vi "Interfaz comunicación chaskas.vi"() -> ()   [LabVIEW 2018]
uses:
  <vilib>/Instr/_visa.llb/VISA Configure Serial Port (Instr).vi
panel:
  out "String":string
  in  "string":string
  in  "Información serial":string
  in  "Interfaz":T1(tab)
  out "Ventana de avisos":string
  out "Nieve disponible":bool
  out "Administrador":bool
  in  "Cerrar Sesión":bool
  in  "Contraseña":string
  out "Usuario actual":string
  in  "Login 2":bool
  in  "Pedido":bool
  in  "Chocolate":bool
  in  "Cereal1":bool
  in  "Cereal 2":bool
  in  "Durazno":bool
  in  "Fresa":bool
  in  "Tamaño de la nieve":enum32{"Chica", "Grande"}(radio)
  out "No se puede borrar:c":string[][](array[string]) caption="transposed array"
  out "Pedido actual":string[][](array[string])
  in  "Mostrar Monitor Serial":bool caption="¿Desea mostrar la información\n Máquina-Interfaz?"
  in  "Bloquear Cereal 2":bool
  in  "Bloquear Cereal 1":bool
  in  "Bloquear chocolate":bool
  in  "Bloquear durazno":bool
  in  "Bloquear fresa":bool
  out "String 2":string
  out "Humedad Relativa Durazno":dbl caption="%Humedad"
  out "Humedad Relativa Fresa":dbl caption="%Humedad"
  out "Humedad Relativa Yogurth":dbl caption="%Humedad"
  out "Temperatura Yogurth":dbl(slide) caption="°C" scale=-20.0..40.0 scale format="%#.1f"
  out "Temperatura fresa":dbl(slide) caption="°C" scale=-20.0..40.0 scale format="%#.1f"
  out "Nivel de Trigo Inflado":dbl(slide) scale=23.0..50.0
  out "Nivel de FrootLoops":dbl(slide) scale=23.0..50.0
  out "Nivel de chocolate":dbl(slide) scale=23.0..50.0
  out "Nivel de yogurth":dbl(slide) scale=23.0..50.0
  out "Nivel de fresa":dbl(slide) scale=23.0..50.0
  in  "Habilitar proceso nieves":bool
  in  "Salir":bool
  out "Nivel de platano":dbl(slide) scale=23.0..50.0
  out "Monitor Serial":string caption="Información Máquina-Interfaz"
  out "Temperatura durazno":dbl(slide) caption="°C" scale=-20.0..40.0 scale format="%#.1f"
  in  "VISA resource name":refnum<visa-resource-name> caption="Puerto de comunicación con la máquina"
  # "Tamaño de la nieve"
  # "1:"
  # "Sabor de la nieve"
  # "2:"
  # "Instrucciones:\n\n1.-Seleccione el tamaño de la nieve.\n2.-Seleccione al menos un sabor, puede ser uno o ambos.\n3.-Seleccione si desea chocolate .\n4.-Seleccione los cereales deseados,\n5.-Cliqueé en \"Realizar Pedido\".\n6.-Confirme datos.\n7.- Por favor espere a que su nieve esté lista\n8.- Disfrute!\n\nVuelva Pronto!:D"
  # "Chocolate"
  # "3:"
  # "Tipos de cereal"
  # "4:"
  # "5:"
  # "Clic para bloquear un ingrediente en caso de que\nse termine"
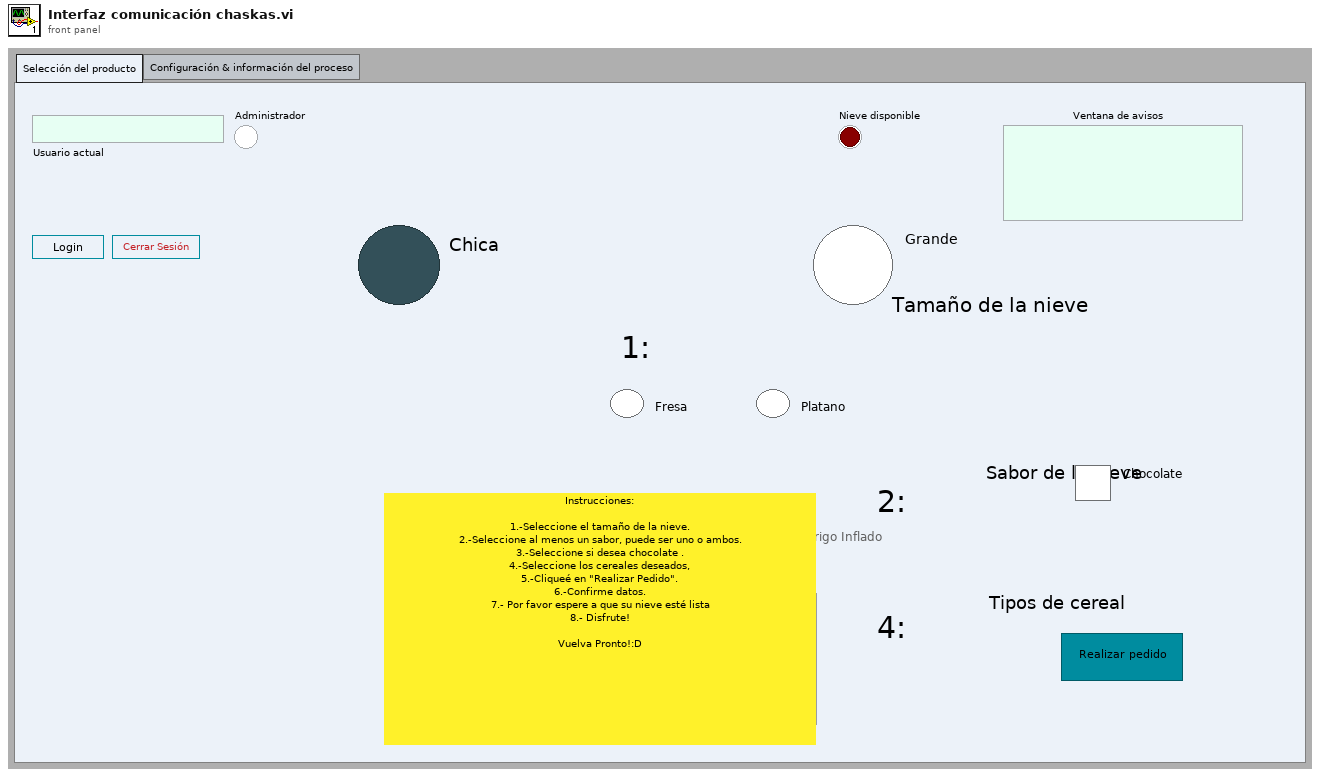
[diagram p1: front panel]
types:
  T1 = enum32{"Selección del producto", "Configuración & información del proceso"}
  T2 = enum8{"Enabled", "Disabled", "Disabled and Grayed Out"}
  T3 = cluster{"Tamaño de la nieve":enum32{"Chica", "Grande"}, "Cereal1":bool, "Chocolate":bool, "Cereal 2":bool, "Durazno":bool, "Fresa":bool}
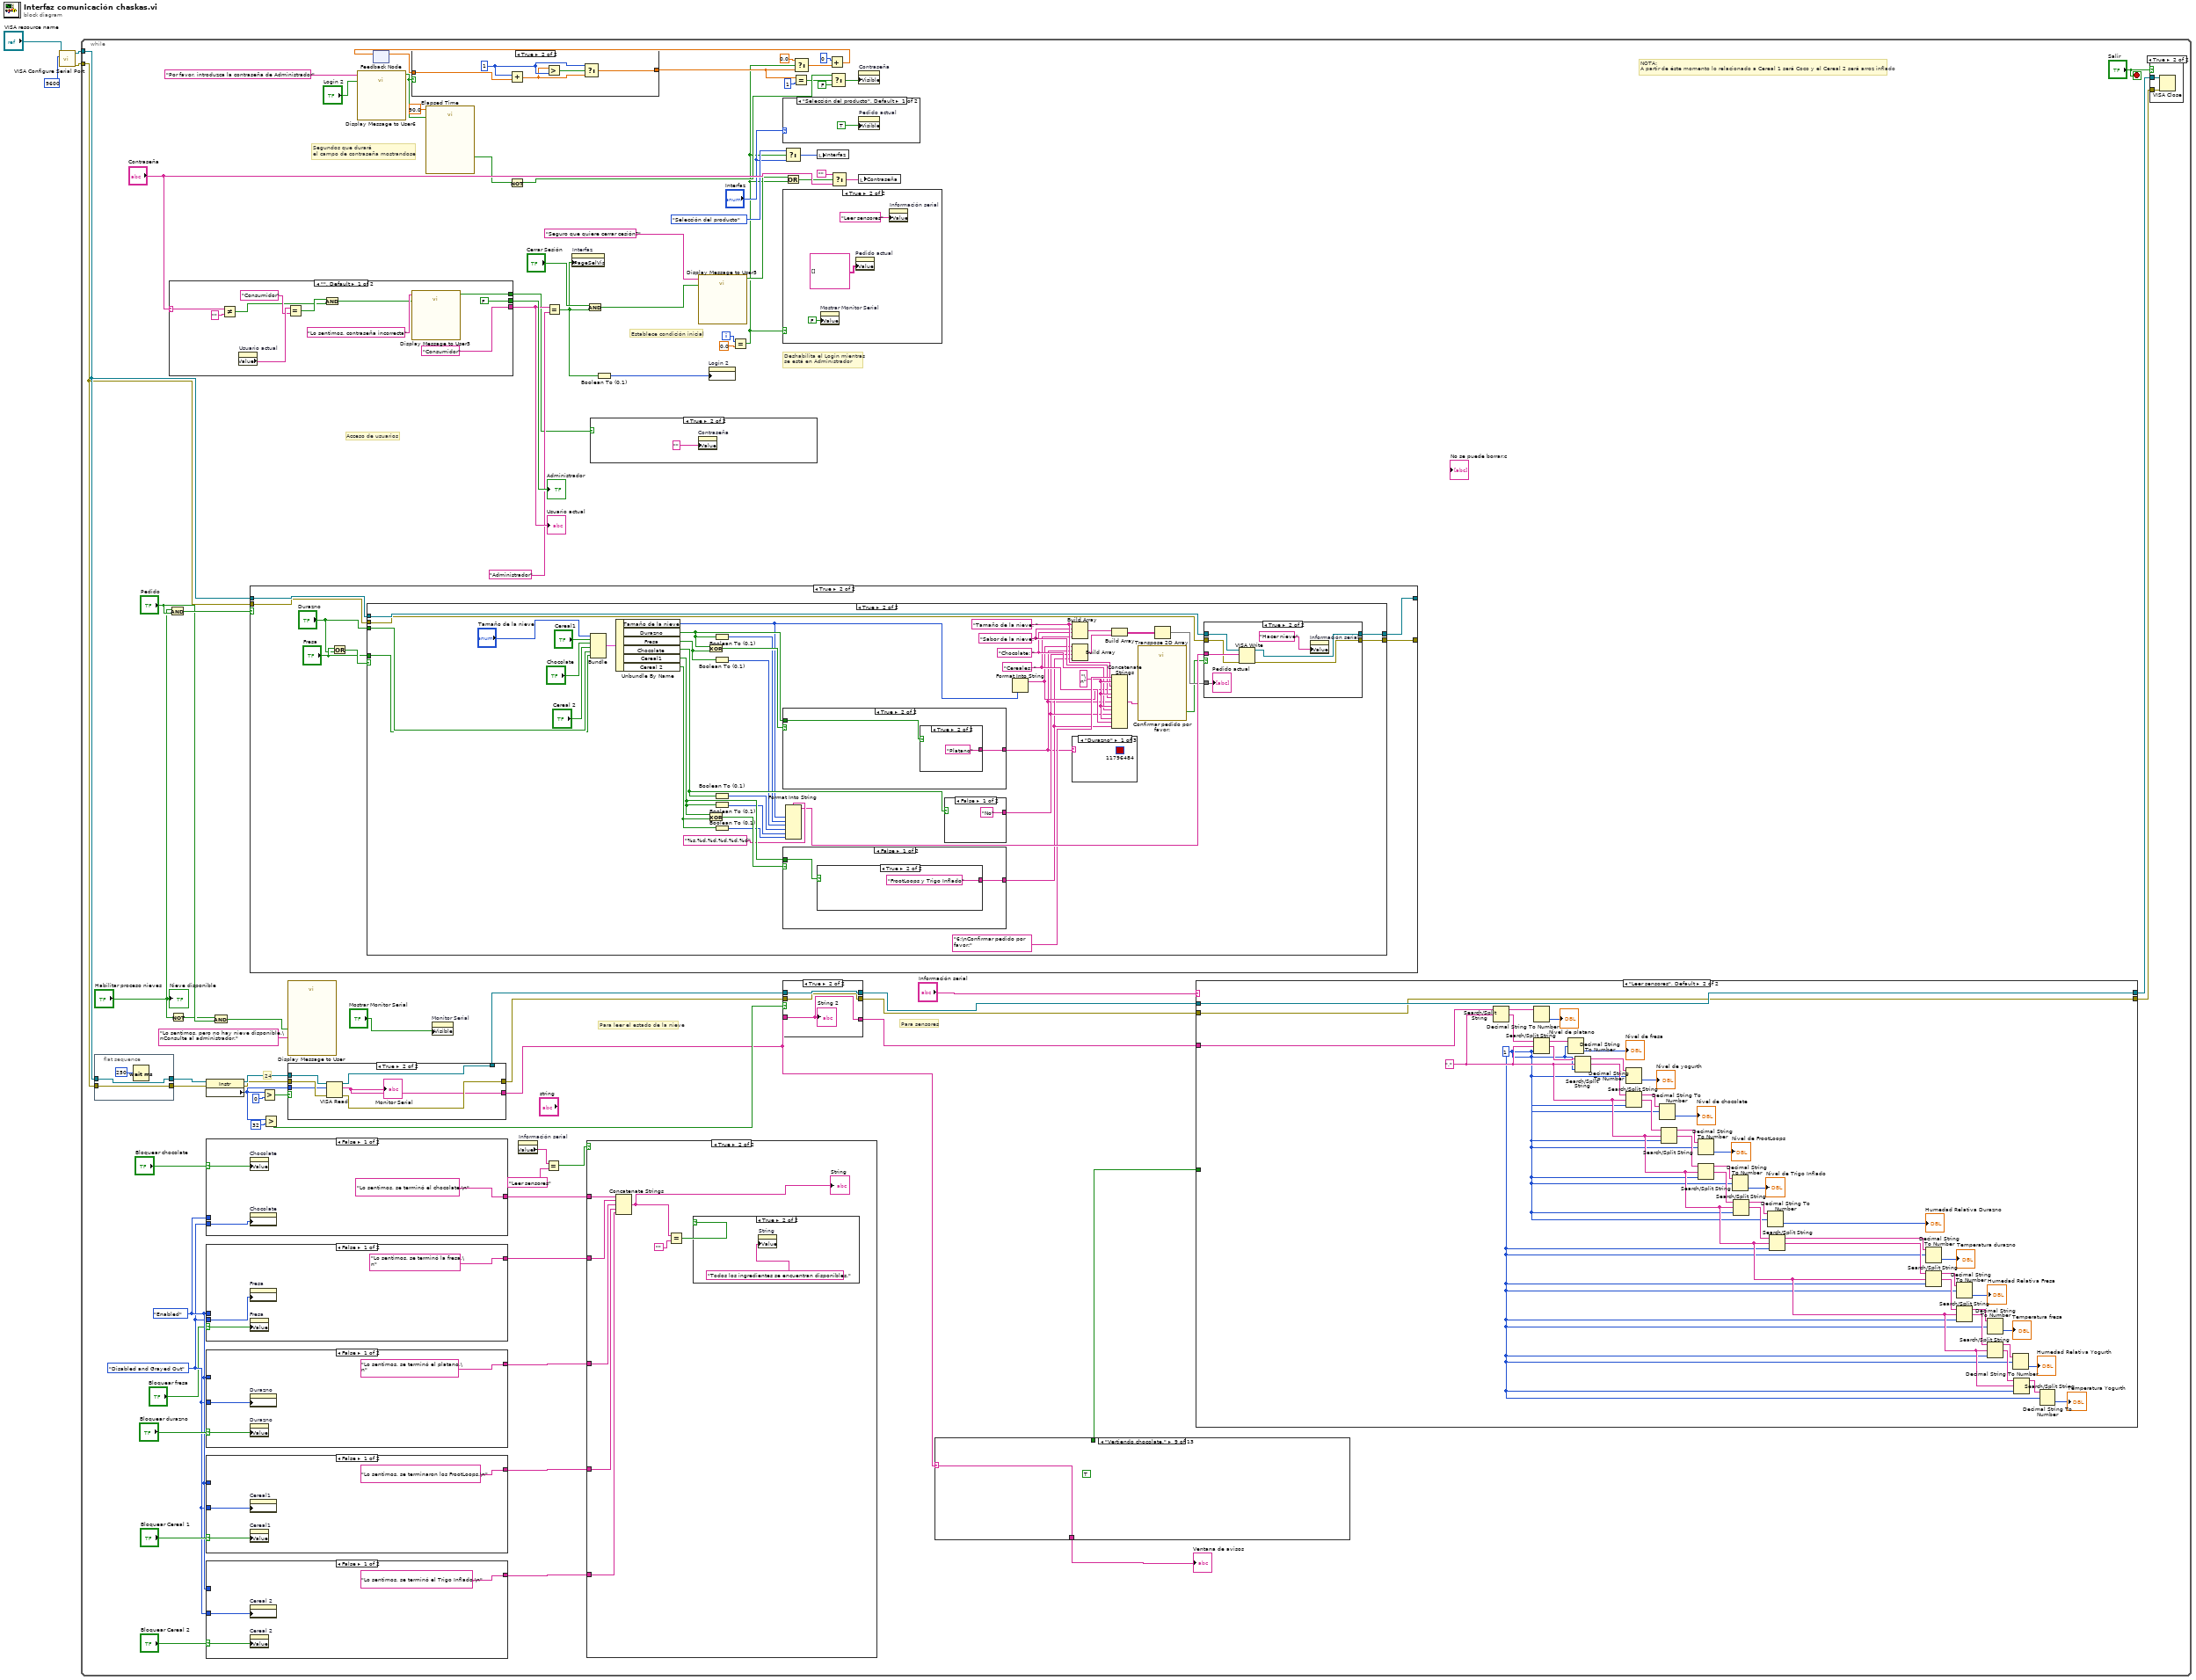
[diagram p0: block diagram]
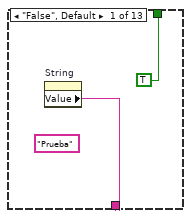
[diagram p2: hidden frame]
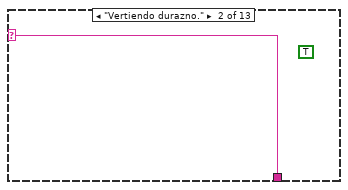
[diagram p3: hidden frame]
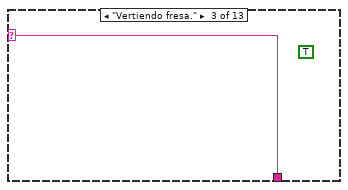
[diagram p4: hidden frame]
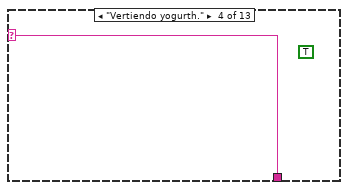
[diagram p5: hidden frame]
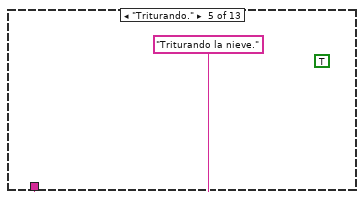
[diagram p6: hidden frame]
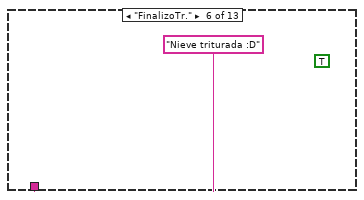
[diagram p7: hidden frame]
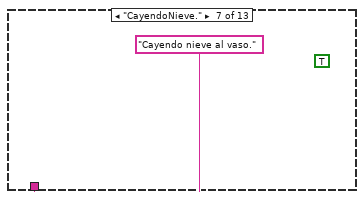
[diagram p8: hidden frame]
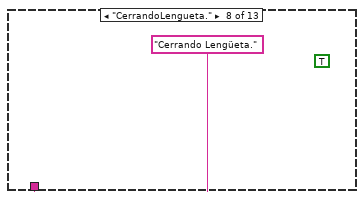
[diagram p9: hidden frame]
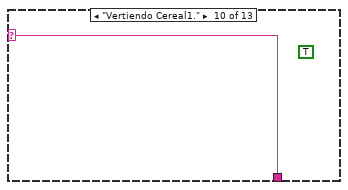
[diagram p10: hidden frame]
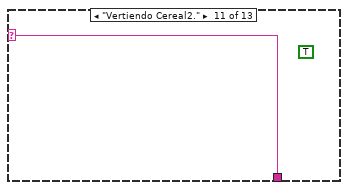
[diagram p11: hidden frame]
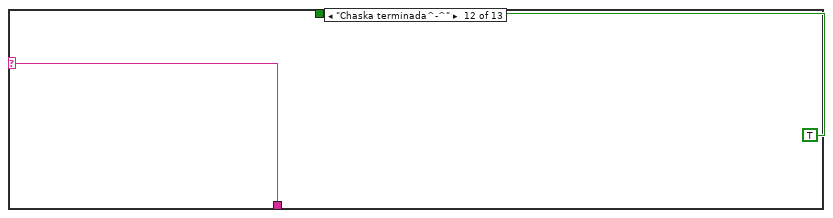
[diagram p12: hidden frame]
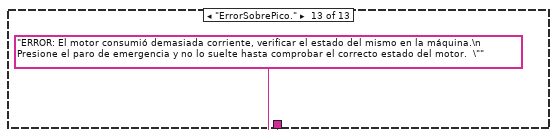
[diagram p13: hidden frame]
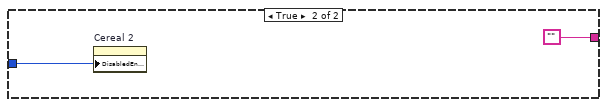
[diagram p17: hidden frame]
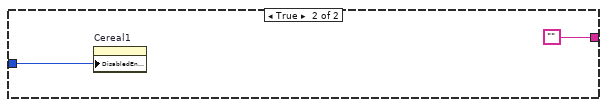
[diagram p18: hidden frame]
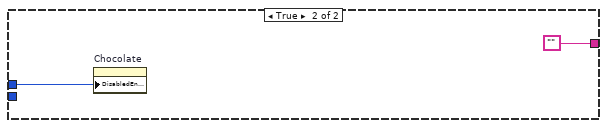
[diagram p19: hidden frame]
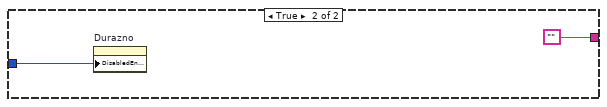
[diagram p20: hidden frame]
diagram:
  n1 = call-poly "VISA Configure Serial Port"("VISA resource name"="VISA resource name", "baud rate (9600)"=u32 9600) -> ("VISA resource name out"=w2:refnum<visa-resource-name>, "error out"=w3:errorcluster)  [unwired: 12 in]
  n2 = while {
    tunnel: w3 -> [w36]
    tunnel: w2 -> [w37]
    i -> [w72]
    stop <- "Salir" stop-if-true
    w21 = T2."Enabled" ("Disabled")
    w20 = T2."Disabled and Grayed Out" ("Disabled")
    # "NOTA:\nA partir de éste momento lo relacionado a Cereal 1 será Coco y el Cereal 2 será arroz inflado"
    # "Segundos que durará \nel campo de contraseña mostrandose"
    # "Acceso de usuarios"
    # "Para leer el estado de la nieve"
    # "Para sensores"
    # "24"
    # "Deshabilita el Login mientras\nse está en Administrador"
    # "Establece condición inicial"
    n3 = flat-sequence {
      tunnel: w37 -> [w204]
      tunnel: [w204] -> w46
      tunnel: [w203] -> w45
      tunnel: w36 -> [w203]
      frame #0 {
        n4 = Wait (ms)(milliseconds to wait=u32 250) -> ()  [unwired: 1 out]
      }
    }
    n5 = case shown="\"\", Default" "Contraseña" {
      selector: "Contraseña" -> [w211 _]
      tunnel: ["Consumidor" "Administrador"] -> w65
      tunnel: [FALSE ("Administrador 2") TRUE ("Administrador 2")] -> w67
      tunnel: [w206 FALSE (":c")] -> w33
      frame "", Default {
        n6 = Not Equal?(x=w211, y="") -> (x != y?=w209:bool)
        n7 = property on="Usuario actual" class="Str"() -> ("Value"=w213:string)  [unwired: 2 in, 2 out]
        n8 = Equal?(x=w213, y="Consumidor") -> (x = y?=w214:bool)
        n9 = And(x=w214, y=w209) -> (x .and. y?=w207:bool)
        n10 = call "Display Message to User3"("Enable"=w207, "Message"="Lo sentimos, contraseña incorrecta") -> (":c"=w206:bool)  [unwired: 8 in, 1 out]
      }
      frame "admin" {
      }
    }
    "Usuario actual" <- w65
    "Administrador" <- w67
    n11 = And(x="Habilitar proceso nieves", y="Pedido") -> (x .and. y?=w85:bool)
    n12 = Not(x="Habilitar proceso nieves") -> (.not. x?=w50:bool)
    n13 = property class="Instr"(reference=w46, error in=w45) -> (reference out=w44:refnum<visa-resource-name>, error out=w43:errorcluster, "Serial Settings:Number of Bytes at Serial Port"=w27:u32)
    n14 = case shown="False" "Bloquear chocolate" {
      selector: "Bloquear chocolate" -> [w124 _]
      tunnel: w21 -> [_ w127]
      tunnel: w20 -> [w125 _]
      tunnel: ["Lo sentimos, se terminó el chocolate.\n" ""] -> w17
      frame False {
        n15 = property on="Chocolate" class="Bool (strict)"("Value"=w124) -> ()  [unwired: 2 in, 2 out]
        n16 = property on="Chocolate" class="Bool (strict)"("DisabledEnum"=w125) -> ()  [unwired: 2 in, 2 out]
      }
      frame True {
        n17 = property on="Chocolate" class="Bool (strict)"("DisabledEnum"=w127) -> ()  [unwired: 2 in, 2 out]
      }
    }
    n18 = case shown="False" "Bloquear fresa" {
      selector: "Bloquear fresa" -> [w134 _]
      tunnel: w20 -> [w135 _]
      tunnel: w21 -> [_ w137]
      tunnel: ["Lo sentimos, se terminó la fresa.\n" ""] -> w16
      frame False {
        n19 = property on="Fresa" class="Bool (strict)"("DisabledEnum"=w135) -> ()  [unwired: 2 in, 2 out]
        n20 = property on="Fresa" class="Bool (strict)"("Value"=w134) -> ()  [unwired: 2 in, 2 out]
      }
      frame True {
        n21 = property on="Fresa" class="Bool (strict)"("DisabledEnum"=w137) -> ()  [unwired: 2 in, 2 out]
      }
    }
    n22 = case shown="False" "Bloquear durazno" {
      selector: "Bloquear durazno" -> [w129 _]
      tunnel: w21 -> [_ w132]
      tunnel: w20 -> [w130 _]
      tunnel: ["Lo sentimos, se terminó el platano.\n" ""] -> w15
      frame False {
        n23 = property on="Durazno" class="Bool (strict)"("DisabledEnum"=w130) -> ()  [unwired: 2 in, 2 out]
        n24 = property on="Durazno" class="Bool (strict)"("Value"=w129) -> ()  [unwired: 2 in, 2 out]
      }
      frame True {
        n25 = property on="Durazno" class="Bool (strict)"("DisabledEnum"=w132) -> ()  [unwired: 2 in, 2 out]
      }
    }
    n26 = case shown="False" "Bloquear Cereal 1" {
      selector: "Bloquear Cereal 1" -> [w119 _]
      tunnel: w21 -> [_ w122]
      tunnel: w20 -> [w120 _]
      tunnel: ["Lo sentimos, se terminaron los FrootLoops.\n" ""] -> w14
      frame False {
        n27 = property on="Cereal1" class="Bool (strict)"("DisabledEnum"=w120) -> ()  [unwired: 2 in, 2 out]
        n28 = property on="Cereal1" class="Bool (strict)"("Value"=w119) -> ()  [unwired: 2 in, 2 out]
      }
      frame True {
        n29 = property on="Cereal1" class="Bool (strict)"("DisabledEnum"=w122) -> ()  [unwired: 2 in, 2 out]
      }
    }
    n30 = case shown="False" "Bloquear Cereal 2" {
      selector: "Bloquear Cereal 2" -> [w114 _]
      tunnel: w21 -> [_ w117]
      tunnel: w20 -> [w115 _]
      tunnel: ["Lo sentimos, se terminó el Trigo Inflado.\n" ""] -> w13
      frame False {
        n31 = property on="Cereal 2" class="Bool (strict)"("DisabledEnum"=w115) -> ()  [unwired: 2 in, 2 out]
        n32 = property on="Cereal 2" class="Bool (strict)"("Value"=w114) -> ()  [unwired: 2 in, 2 out]
      }
      frame True {
        n33 = property on="Cereal 2" class="Bool (strict)"("DisabledEnum"=w117) -> ()  [unwired: 2 in, 2 out]
      }
    }
    n34 = And(x=w50, y="Pedido") -> (x .and. y?=w48:bool)
    n35 = case shown="True" w85 {
      tunnel: w37 -> [w229 w233]
      tunnel: w36 -> [w228 w232]
      tunnel: [w229 w231] -> _
      tunnel: [w228 w230] -> _
      frame False {
      }
      frame True {
        n36 = Or(x="Fresa", y="Durazno") -> (x .or. y?=w236:bool)
        n37 = case shown="True" w236 {
          tunnel: "Fresa" -> [_ w277]
          tunnel: "Durazno" -> [_ w278]
          tunnel: w233 -> [w238 w259]
          tunnel: w232 -> [w237 w249]
          tunnel: [w238 w248] -> w231
          tunnel: [w237 w247] -> w230
          frame False {
            n38 = call "Display Message to User2"("Message"="Por favor, seleccione al menos un sabor de fruta.") -> ()  [unwired: 9 in, 2 out]
          }
          frame True {
            w253 = "Cereales: " ("string")
            w254 = "Chocolate: " ("string")
            w255 = "Sabor de la nieve: " ("string")
            w257 = "\n" ("string")
            w256 = "Tamaño de la nieve: " ("string")
            n39 = Bundle("Tamaño de la nieve"="Tamaño de la nieve", "Cereal1"="Cereal1", "Chocolate"="Chocolate", "Cereal 2"="Cereal 2", "Durazno"=w278, "Fresa"=w277) -> (w276:T3)  [unwired: 1 in]
            n40 = Unbundle By Name(w276) -> ("Tamaño de la nieve"=w262:enum32{"Chica", "Grande"}, "Durazno"=w272:bool, "Fresa"=w271:bool, "Chocolate"=w270:bool, "Cereal1"=w269:bool, "Cereal 2"=w268:bool)
            n41 = Exclusive Or(1:w271, 2:w272) -> (0:w275:bool)
            n42 = Exclusive Or(1:w268, 2:w269) -> (0:w274:bool)
            n43 = Boolean To (0,1)(Boolean=w272) -> (0, 1=w267:i16)
            n44 = Boolean To (0,1)(Boolean=w271) -> (0, 1=w266:i16)
            n45 = Boolean To (0,1)(Boolean=w270) -> (0, 1=w265:i16)
            n46 = Boolean To (0,1)(Boolean=w269) -> (0, 1=w264:i16)
            n47 = Boolean To (0,1)(Boolean=w268) -> (0, 1=w263:i16)
            n48 = case shown="True" w275 {
              tunnel: [w300 w304] -> w243
              tunnel: w272 -> [w299 w303]
              frame False {
                n49 = case shown="True" w299 {
                  tunnel: [" " "Fresa y Platano"] -> w300
                  frame False {
                  }
                  frame True {
                  }
                }
              }
              frame True {
                n50 = case shown="True" w303 {
                  tunnel: ["Fresa" "Platano"] -> w304
                  frame False {
                  }
                  frame True {
                  }
                }
              }
            }
            n51 = case shown="False" w274 {
              tunnel: w269 -> [w292 w296]
              tunnel: [w291 w295] -> w250
              frame False {
                n52 = case shown="True" w292 {
                  tunnel: ["Ninguno" "FrootLoops y Trigo Inflado"] -> w291
                  frame False {
                  }
                  frame True {
                  }
                }
              }
              frame True {
                n53 = case shown="False" w296 {
                  tunnel: ["Trigo Inflado" "FrootLoops"] -> w295
                  frame False {
                  }
                  frame True {
                  }
                }
              }
            }
            n54 = Format Into String(format string="%s,%d,%d,%d,%d,%d", w262, w267, w266, w265, w264, w263) -> (resulting string=w260:string)  [unwired: 2 in, 1 out]
            n55 = case shown="False" w270 {
              tunnel: ["No" "Sí"] -> w251
              frame False {
              }
              frame True {
              }
            }
            n56 = Format Into String(w262) -> (resulting string=w252:string)  [unwired: 3 in, 1 out]
            n57 = Build Array(w256, w255, w254, w253) -> (w246:string[])
            n58 = Build Array(w252, w243, w251, w250) -> (w245:string[])
            n59 = case shown="\"Durazno\"" w243 {
              frame "Durazno" {
                (unwired) u32 11796484
              }
              frame "Fresa" {
              }
              frame "Fresa y Durazno", Default {
              }
            }
            n60 = Build Array(w246, w245) -> (w244:string[][])
            n61 = Concatenate Strings("6:\nConfirmar pedido por favor:" ("string"), w257, w256, w252, w257, w255, w243, w257, w254, w251, w257, w253, w250) -> (w241:string)
            n62 = call "Confirmar pedido por favor:"("Message"=w241) -> ("Está bien"=w240:bool)  [unwired: 9 in, 1 out]
            n63 = Transpose 2D Array(2D array=w244) -> (transposed array=w242:string[][])
            n64 = case shown="True" w240 {
              tunnel: w260 -> [_ w290]
              tunnel: w259 -> [w283 w289]
              tunnel: w249 -> [w282 w288]
              tunnel: [w283 w287] -> w248
              tunnel: [w282 w286] -> w247
              tunnel: w242 -> [_ w284]
              frame False {
              }
              frame True {
                n65 = VISA Write(VISA resource name=w289, write buffer=w290, error in (no error)=w288) -> (VISA resource name out=w287:refnum<visa-resource-name>, error out=w286:errorcluster)  [unwired: 1 out]
                n66 = property on="Información serial" class="Str"("Value"="Hacer nieve") -> ()  [unwired: 2 in, 2 out]
                "Pedido actual" <- w284
              }
            }
          }
        }
      }
    }
    n67 = Greater?(x=w27, y=u32 0) -> (0:w42:bool)
    n68 = Greater?(x=w27, y=u32 32) -> (0:w31:bool)
    n69 = call "Display Message to User"("Enable"=w48, "Message"="Lo sentimos, pero no hay nieve disponible.\nConsulte al administrador.") -> ()  [unwired: 8 in, 2 out]
    n70 = case shown="True" w42 {
      tunnel: w44 -> [w151 w157]
      tunnel: [w151 w156] -> w29
      tunnel: w43 -> [w150 w155]
      tunnel: w27 -> [_ w154]
      tunnel: [w150 w153] -> w28
      tunnel: [w149 w152] -> w5
      frame False {
        n71 = property on="Monitor Serial" class="Str"() -> ("Value"=w149:string)  [unwired: 2 in, 2 out]
      }
      frame True {
        n72 = VISA Read(VISA resource name=w157, byte count=w154, error in (no error)=w155) -> (VISA resource name out=w156:refnum<visa-resource-name>, read buffer=w152:string, error out=w153:errorcluster)  [unwired: 1 out]
        "Monitor Serial" <- w152
      }
    }
    n73 = call "Display Message to User6"("Enable"="Login 2", "Message"="Por favor, introduzca la contraseña de Administrador") -> ("Claro"=w34:bool)  [unwired: 8 in, 1 out]
    n74 = feedback #1() -> (w74:dbl)  [unwired: 1 in]
    n75 = case shown="True" w34 {
      tunnel: [w221 w223] -> w69
      tunnel: w74 -> [w220 w227]
      frame False {
        n76 = Add(x=0, y=w220) -> (x+y=w221:dbl)
      }
      frame True {
        w225 = 1 ("x")
        n77 = Add(x=w225, y=w227) -> (x+y=w224:dbl)
        n78 = Greater?(x=w224, y=w225) -> (0:w226:bool)
        n79 = Select(t=w225, s=w226, f=w224) -> (s? t:f=w223:dbl)
      }
    }
    n80 = call "Elapsed Time"("Time Target (s)"=90.0, "Reset"=w34) -> ("Time has Elapsed"=w81:bool)  [unwired: 10 in, 7 out]
    n81 = property on="Monitor Serial" class="Str"("Visible"="Mostrar Monitor Serial") -> ()  [unwired: 2 in, 2 out]
    n82 = Not(x=w81) -> (.not. x?=w80:bool)
    n83 = property on="Información serial" class="Str"() -> ("Value"=w10:string)  [unwired: 2 in, 2 out]
    n84 = Equal?(x=w10, y="Leer sensores") -> (x = y?=w8:bool)
    n85 = Equal?(x=w65, y="Administrador") -> (x = y?=w55:bool)
    n86 = property on="Interfaz" class="TabCtl (strict)"("PageSelVis"=w55) -> ()  [unwired: 2 in, 2 out]
    n87 = case shown="True" w8 {
      tunnel: w17 -> [_ w108]
      tunnel: w16 -> [_ w107]
      tunnel: w15 -> [_ w106]
      tunnel: w14 -> [_ w105]
      tunnel: w13 -> [_ w104]
      frame False {
      }
      frame True {
        n88 = Concatenate Strings(w108, w107, w106, w105, w104) -> (w101:string)
        "String" <- w101
        n89 = Equal?(x=w101, y="") -> (x = y?=w102:bool)
        n90 = case shown="True" w102 {
          frame False {
          }
          frame True {
            n91 = property on="String" class="Str"("Value"="Todos los ingredientes se encuentran disponibles." ("Ingredientes faltantes")) -> ()  [unwired: 2 in, 2 out]
          }
        }
      }
    }
    n92 = And(x="Cerrar Sesión", y=w55) -> (x .and. y?=w66:bool)
    n93 = case shown="True" w33 {
      frame False {
      }
      frame True {
        n94 = property on="Contraseña" class="Str"("Value"="" ("Contraseña")) -> ()  [unwired: 2 in, 2 out]
      }
    }
    n95 = Boolean To (0,1)(Boolean=w55) -> (0, 1=w60:i16)
    n96 = call "Display Message to User5"("Enable"=w66, "Message"="Seguro que quiere cerrar cesión?") -> ("Sí"=w57:bool)  [unwired: 8 in, 1 out]
    n97 = property on="Login 2" class="Bool"("DisabledEnum"=w60) -> ()  [unwired: 2 in, 2 out]
    n98 = Equal?(x=w72, y=0.0) -> (x = y?=w12:bool)
    n99 = case shown="\"Selección del producto\", Default" "Interfaz" {
      frame "Selección del producto", Default {
        n100 = property on="Pedido actual" class="Arr (strict)"("Visible"=TRUE) -> ()  [unwired: 2 in, 2 out]
      }
      frame "Configuración & información del proceso" {
        n101 = property on="No se puede borrar:c" class="Arr (strict)"("Visible"=FALSE) -> ()  [unwired: 2 in, 2 out]
      }
    }
    n102 = case shown="True" w12 {
      frame False {
      }
      frame True {
        n103 = property on="Mostrar Monitor Serial" class="Bool (strict)"("Value"=FALSE ("Mostrar Monitor Serial")) -> ()  [unwired: 2 in, 2 out]
        n104 = property on="Pedido actual" class="Arr (strict)"("Value"=string[][] []) -> ()  [unwired: 2 in, 2 out]
        n105 = property on="Información serial" class="Str"("Value"="Leer sensores" ("String")) -> ()  [unwired: 2 in, 2 out]
      }
    }
    n106 = case shown="True" w31 {
      tunnel: [w138 w143] -> w30
      tunnel: w29 -> [w140 w142]
      tunnel: w28 -> [w139 w141]
      tunnel: [w140 w142] -> w26
      tunnel: [w139 w141] -> w25
      tunnel: w5 -> [_ w143]
      frame False {
        n107 = property on="String 2" class="Str"() -> ("Value"=w138:string)  [unwired: 2 in, 2 out]
      }
      frame True {
        "String 2" <- w143
      }
    }
    n108 = Select(t=T1."Selección del producto" ("Interfaz"), s=w12, f="Interfaz") -> (s? t:f=w54:T1)
    n109 = Or(x=w57, y=w12) -> (x .or. y?=w56:bool)
    n110 = Equal?(x=w69, y=1) -> (x = y?=w62:bool)
    n111 = Select(t=0.0, s=w12, f=w69) -> (s? t:f=w70:dbl)
    n112 = local write "Interfaz"(w54) -> ()
    n113 = Add(x=0, y=w70) -> (x+y=w75:dbl)
    n114 = feedback-in #1(w75) -> ()
    n115 = Select(t=w80, s=w62, f=FALSE) -> (s? t:f=w79:bool)
    n116 = Select(t="", s=w56, f="Contraseña") -> (s? t:f=w83:string)
    n117 = property on="Contraseña" class="Str"("Visible"=w79) -> ()  [unwired: 2 in, 2 out]
    n118 = local write "Contraseña"(w83) -> ()
    n119 = case shown="\"Vertiendo chocolate.\"" w5 {
      selector: w5 -> [_ w88 w89 w90 _ _ _ _ w95 w96 w97 w99 _]
      tunnel: [w86 w88 w89 w90 "Triturando la nieve." ("Comunicacion con el cliente") "Nieve triturada :D" ("Comunicacion con el cliente") "Cayendo nieve al vaso." ("Comunicacion con el cliente") "Cerrando Lengüeta." ("Comunicacion con el cliente") w95 w96 w97 w99 "ERROR: El motor consumió demasiada corriente, verificar el estado del mismo en la máquina.\n Presione el paro de emergencia y no lo suelte hasta comprobar el correcto estado del motor.  \"" ("Comunicacion con el cliente")] -> w7
      tunnel: [TRUE _ _ _ _ _ _ _ _ _ _ TRUE _] -> w6
      frame "False", Default {
        (unwired) "Prueba"
        n120 = property on="String" class="Str"() -> ("Value"=w86:string)  [unwired: 2 in, 2 out]
      }
      frame "Vertiendo durazno." {
        (unwired) TRUE
      }
      frame "Vertiendo fresa." {
        (unwired) TRUE
      }
      frame "Vertiendo yogurth." {
        (unwired) TRUE
      }
      frame "Triturando." {
        (unwired) TRUE
      }
      frame "FinalizoTr." {
        (unwired) TRUE
      }
      frame "CayendoNieve." {
        (unwired) TRUE
      }
      frame "CerrandoLengueta." {
        (unwired) TRUE
      }
      frame "Vertiendo chocolate." {
        (unwired) TRUE
      }
      frame "Vertiendo Cereal1." {
        (unwired) TRUE
      }
      frame "Vertiendo Cereal2." {
        (unwired) TRUE
      }
      frame "Chaska terminada^-^" {
      }
      frame "ErrorSobrePico." {
      }
    }
    "Ventana de avisos" <- w7
    n121 = case shown="\"Leer sensores\", Default" "Información serial" {
      tunnel: [w159 w176] -> w39
      tunnel: [w160 w163] -> w40
      tunnel: w26 -> [w159 w176]
      tunnel: w30 -> [_ w175]
      tunnel: w25 -> [w160 w163]
      tunnel: w6 -> [w158 _]
      frame "Hacer nieve" {
        # "Corregir los if para poder ver en qué parte del proceso vamos"
        n122 = case shown="True" w158 {
          frame False {
          }
          frame True {
            n123 = flat-sequence {
              frame #0 {
                n124 = Wait (ms)(milliseconds to wait=u32 3000) -> ()  [unwired: 1 out]
              }
              frame #1 {
                n125 = property on="Información serial" class="Str"("Value"="Leer sensores" ("String")) -> ()  [unwired: 2 in, 2 out]
              }
            }
          }
        }
      }
      frame "Leer sensores", Default {
        w164 = 1 ("offset (0)")
        w177 = "," ("search string/char (-)")
        n126 = Search/Split String(string=w175, search string/char (-)=w177) -> (substring before match=w202:string, match + rest of string=w201:string)  [unwired: 1 in, 1 out]
        n127 = Decimal String To Number(string=w202) -> (number=→"Nivel de platano":i32)  [unwired: 2 in, 1 out]
        n128 = Search/Split String(string=w201, search string/char (-)=w177, offset (0)=w164) -> (substring before match=w200:string, match + rest of string=w198:string)  [unwired: 1 out]
        n129 = Decimal String To Number(string=w200, offset=w164) -> (number=→"Nivel de fresa":i32)  [unwired: 1 in, 1 out]
        n130 = Search/Split String(string=w198, search string/char (-)=w177, offset (0)=w164) -> (substring before match=w199:string, match + rest of string=w196:string)  [unwired: 1 out]
        n131 = Decimal String To Number(string=w199, offset=w164) -> (number=→"Nivel de yogurth":i32)  [unwired: 1 in, 1 out]
        n132 = Search/Split String(string=w196, search string/char (-)=w177, offset (0)=w164) -> (substring before match=w193:string, match + rest of string=w195:string)  [unwired: 1 out]
        n133 = Decimal String To Number(string=w193, offset=w164) -> (number=→"Nivel de chocolate":i32)  [unwired: 1 in, 1 out]
        n134 = Search/Split String(string=w195, search string/char (-)=w177, offset (0)=w164) -> (substring before match=w192:string, match + rest of string=w194:string)  [unwired: 1 out]
        n135 = Decimal String To Number(string=w192, offset=w164) -> (number=→"Nivel de FrootLoops":i32)  [unwired: 1 in, 1 out]
        n136 = Search/Split String(string=w194, search string/char (-)=w177, offset (0)=w164) -> (substring before match=w191:string, match + rest of string=w188:string)  [unwired: 1 out]
        n137 = Decimal String To Number(string=w191, offset=w164) -> (number=→"Nivel de Trigo Inflado":i32)  [unwired: 1 in, 1 out]
        n138 = Search/Split String(string=w188, search string/char (-)=w177, offset (0)=w164) -> (substring before match=w187:string, match + rest of string=w186:string)  [unwired: 1 out]
        n139 = Decimal String To Number(string=w187, offset=w164) -> (number=→"Humedad Relativa Durazno":i32)  [unwired: 1 in, 1 out]
        n140 = Search/Split String(string=w186, search string/char (-)=w177, offset (0)=w164) -> (substring before match=w189:string, match + rest of string=w182:string)  [unwired: 1 out]
        n141 = Decimal String To Number(string=w189, offset=w164) -> (number=→"Temperatura durazno":i32)  [unwired: 1 in, 1 out]
        n142 = Search/Split String(string=w182, search string/char (-)=w177, offset (0)=w164) -> (substring before match=w183:string, match + rest of string=w184:string)  [unwired: 1 out]
        n143 = Decimal String To Number(string=w183, offset=w164) -> (number=→"Humedad Relativa Fresa":i32)  [unwired: 1 in, 1 out]
        n144 = Search/Split String(string=w184, search string/char (-)=w177, offset (0)=w164) -> (substring before match=w185:string, match + rest of string=w179:string)  [unwired: 1 out]
        n145 = Decimal String To Number(string=w185, offset=w164) -> (number=→"Temperatura fresa":i32)  [unwired: 1 in, 1 out]
        n146 = Search/Split String(string=w179, search string/char (-)=w177, offset (0)=w164) -> (substring before match=w178:string, match + rest of string=w180:string)  [unwired: 1 out]
        n147 = Decimal String To Number(string=w178, offset=w164) -> (number=→"Humedad Relativa Yogurth":i32)  [unwired: 1 in, 1 out]
        n148 = Search/Split String(string=w180, search string/char (-)=w177, offset (0)=w164) -> (substring before match=w181:string)  [unwired: 2 out]
        n149 = Decimal String To Number(string=w181, offset=w164) -> (number=→"Temperatura Yogurth":i32)  [unwired: 1 in, 1 out]
      }
    }
    n150 = case shown="True" "Salir" {
      tunnel: w40 -> [_ w146]
      tunnel: w39 -> [_ w145]
      frame False {
      }
      frame True {
        n151 = VISA Close(VISA resource name=w145, error in (no error)=w146) -> ()  [unwired: 1 out]
      }
    }
    "Nieve disponible" <- "Habilitar proceso nieves"
  }
